vi "AnalogOutput-Drive.vi"(8 "error in":errorcluster, 9 "Waveform":waveform(dbl)={"t0"=timestamp(0 s since 1904-01-01), "dt"=0.0, "Y"=[]}, 10 "Timestamp line":tag, 11 "Line":tag) -> (0 "error out":errorcluster)   [LabVIEW 2015]
doc: "Drives an analog output line.\n\nLine:\n Analog output line\nTimestamp line: \n Pretty self-explanatory.\n Empty or unwired for no timestamp\nWaveform:\n Analog waveform to output\n\nTiming warnings: The timestamp pulse is 2 waveform samples long. That comes out to 20 us at a 100 kHz sample rate.\n\nAlso, it takes about 20 ms from calling this code to actual waveform generation. I don't know how to make that any faster.\n\nFinally, this code doesn't return until the analog output stops."
uses:
  <vilib>/DAQmx/write.llb/DAQmx Write (Digital Wfm 1Chan NSamp).vi
  <vilib>/DAQmx/write.llb/DAQmx Write (Analog Wfm 1Chan NSamp).vi
  <vilib>/Waveform/WDTOps.llb/WDT Number of Waveform Samples DBL.vi
  <vilib>/DAQmx/create/channels.llb/DAQmx Create Channel (DO-Digital Output).vi
  <vilib>/Waveform/DWDTOps.llb/DWDT Boolean Array to Digital.vi
  <vilib>/DAQmx/configure/timing.llb/DAQmx Timing (Sample Clock).vi
  <vilib>/Waveform/DWDTOps.llb/DWDT Uncompress Digital.vi
  <vilib>/DAQmx/miscellaneous.llb/DAQmx Fill In Error Info.vi
  <vilib>/DAQmx/create/channels.llb/DAQmx Create Channel (AO-Voltage-Basic).vi
  <resource>/objmgr/daqmx.rc
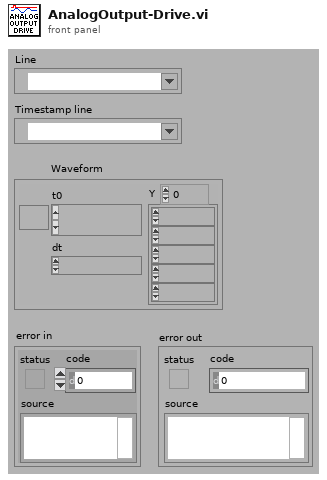
[diagram p1: front panel]
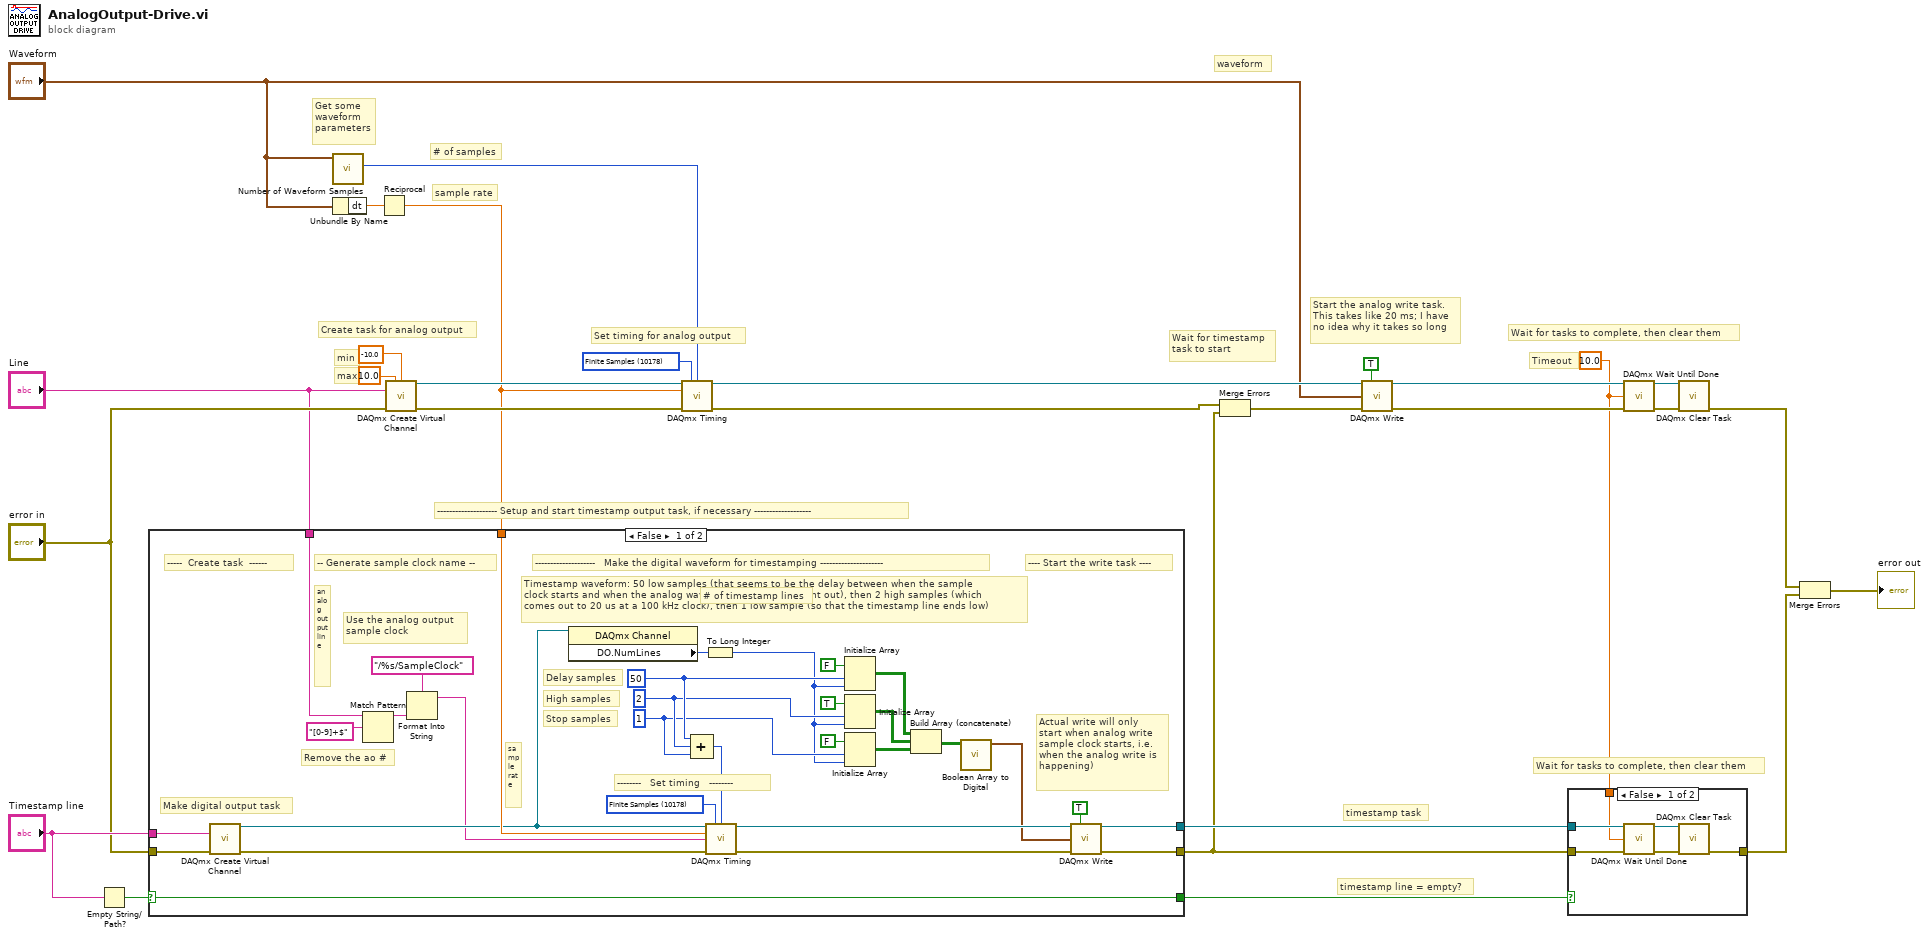
[diagram p0: block diagram]
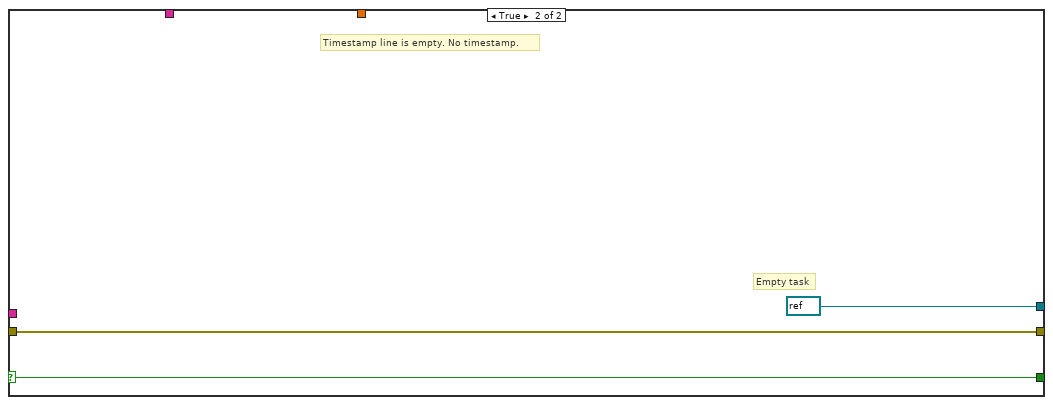
[diagram p3: hidden frame]
diagram:
  w6 = 10.0 ("timeout (sec)")
  w25 = 10178 items=["Finite Samples"=10178, "Continuous Samples"=10123] ("sample mode")
  # "timestamp line = empty?"
  # "timestamp task"
  # "waveform"
  # "Wait for tasks to complete, then clear them"
  # "Wait for tasks to complete, then clear them"
  # "Timeout"
  # "Start the analog write task.\nThis takes like 20 ms; I have\nno idea why it takes so long"
  # "Wait for timestamp\ntask to start"
  # "-------------------- Setup and start timestamp output task, if necessary -------------------"
  # "Get some\nwaveform\nparameters"
  # "# of samples"
  # "sample rate"
  # "Set timing for analog output"
  # "Create task for analog output"
  # "max"
  # "min"
  n1 = Empty String/Path?(string/path="Timestamp line") -> (empty?=w18:bool)
  n2 = call-poly <vilib>:"Number of Waveform Samples.vi"("waveform in"="Waveform") -> ("number of samples"=w22:i32)  [unwired: 8 in, 2 out]
  n3 = Unbundle By Name("Waveform") -> ("dt"=w28:dbl)
  n4 = Reciprocal(x=w28) -> (1/x=w19:dbl)
  n5 = case shown="False" w18 {
    selector: w18 -> [w34 w61]
    tunnel: "Timestamp line" -> [w59 _]
    tunnel: "error in" -> [w58 w62]
    tunnel: w19 -> [w55 _]
    tunnel: [w35 w62] -> w7
    tunnel: [w34 w61] -> w5
    tunnel: [w36 refnum<k21> refnum ("task out")] -> w8
    tunnel: "Line" -> [w32 _]
    frame False {
      w48 = 1 ("samples per channel")
      w49 = 2 ("samples per channel")
      w50 = 50 ("samples per channel")
      w57 = 10178 items=["Finite Samples"=10178, "Continuous Samples"=10123] ("sample mode")
      # "analog output line"
      # "sample rate"
      # "Use the analog output \nsample clock"
      # "-- Generate sample clock name --"
      # "Remove the ao #"
      # "Make digital output task"
      # "---- Start the write task ----"
      # "Timestamp waveform: 50 low samples (that seems to be the delay between when the sample \nclock starts and when the analog waveform actually gets sent out), then 2 high samples (which\ncomes out to 20 us at a 100 kHz clock), then 1 low sample (so that the timestamp line ends low)"
      # "Actual write will only\nstart when analog write\nsample clock starts, i.e.\nwhen the analog write is\nhappening)"
      # "--------------------   Make the digital waveform for timestamping ---------------------"
      # "# of timestamp lines"
      # "Stop samples"
      # "--------   Set timing   --------"
      # "-----  Create task  ------"
      # "High samples"
      # "Delay samples"
      n6 = call-poly <vilib>:"DAQmx Create Virtual Channel.vi"("lines"=w59, "error in"=w58) -> ("task out"=w38:refnum<k21>, "error out"=w56:errorcluster)  [unwired: 12 in]
      n7 = Match Pattern(string=w32, regular expression="[0-9]+$") -> (before substring=w30:string)  [unwired: 1 in, 3 out]
      n8 = Format Into String(format string="/%s/SampleClock", w30) -> (resulting string=w29:string)  [unwired: 2 in, 1 out]
      n9 = property class="DAQmx Channel"(reference=w38) -> ("DO.NumLines"=w40:u32)  [unwired: 1 in, 2 out]
      n10 = Compound Arithmetic op=unknown(w50, w49, w48) -> (w54:i32)
      n11 = To Long Integer(number=w40) -> (32bit integer=w39:i32)
      n12 = call-poly <vilib>:"DAQmx Timing.vi"("task/channels in"=w38, "sample mode"=w57, "samples per channel"=w54, "rate"=w55, "source"=w29, "error in"=w56) -> ("task out"=w43:refnum<k21>, "error out"=w42:errorcluster)  [unwired: 8 in]
      n13 = Initialize Array(FALSE ("element"), w50, w39) -> (w45:bool[][])
      n14 = Initialize Array(TRUE ("element"), w49, w39) -> (w46:bool[][])
      n15 = Initialize Array(FALSE ("element"), w48, w39) -> (w47:bool[][])
      n16 = Build Array (concatenate)(w45, w46, w47) -> (w44:bool[][])
      n17 = call-poly <vilib>:"Boolean Array to Digital.vi"("boolean array"=w44) -> ("digital waveform"=w41:digitalwaveform)  [unwired: 9 in, 1 out]
      n18 = call-poly <vilib>:"DAQmx Write.vi"("task/channels in"=w43, "auto start"=TRUE, "data"=w41, "error in"=w42) -> ("task out"=w36:refnum<k21>, "error out"=w35:errorcluster)  [unwired: 9 in, 1 out]
    }
    frame True {
      # "Empty task"
      # "Timestamp line is empty. No timestamp."
    }
  }
  n19 = call-poly <vilib>:"DAQmx Create Virtual Channel.vi"("maximum value"=10.0, "minimum value"=-10.0, "physical channels"="Line", "error in"="error in") -> ("task out"=w24:refnum<k21>, "error out"=w23:errorcluster)  [unwired: 10 in]
  n20 = call-poly <vilib>:"DAQmx Timing.vi"("task/channels in"=w24, "sample mode"=w25, "samples per channel"=w22, "rate"=w19, "error in"=w23) -> ("task out"=w16:refnum<k21>, "error out"=w17:errorcluster)  [unwired: 9 in]
  n21 = Merge Errors(w17, w7) -> (w14:errorcluster)
  n22 = call-poly <vilib>:"DAQmx Write.vi"("task/channels in"=w16, "auto start"=TRUE, "data"="Waveform", "error in"=w14) -> ("task out"=w9:refnum<k21>, "error out"=w10:errorcluster)  [unwired: 9 in, 1 out]
  n23 = case shown="False" w5 {
    tunnel: w8 -> [w66 _]
    tunnel: w7 -> [w65 w69]
    tunnel: w6 -> [w64 _]
    tunnel: [w63 w69] -> w2
    frame False {
      n24 = call <vilib>:"DAQmx Wait Until Done.vi"("task/channels in"=w66, "timeout (sec)"=w64, "error in"=w65) -> ("task out"=w68:refnum<k21>, "error out"=w67:errorcluster)  [unwired: 11 in]
      n25 = call <vilib>:"DAQmx Clear Task.vi"("task in"=w68, "error in"=w67) -> ("error out"=w63:errorcluster)  [unwired: 13 in]
    }
    frame True {
    }
  }
  n26 = call <vilib>:"DAQmx Wait Until Done.vi"("task/channels in"=w9, "timeout (sec)"=w6, "error in"=w10) -> ("task out"=w12:refnum<k21>, "error out"=w11:errorcluster)  [unwired: 11 in]
  n27 = call <vilib>:"DAQmx Clear Task.vi"("task in"=w12, "error in"=w11) -> ("error out"=w3:errorcluster)  [unwired: 13 in]
  n28 = Merge Errors(w3, w2) -> (→"error out":errorcluster)
